vi "Keep Alive Interval.vi"(8 "error in (no error)":errorcluster, 9 "Connection Name":string, 11 "Keep Alive Interval (s)":i32) -> (0 "error out":errorcluster)   [LabVIEW 2018, in "LabSFTP.lvlib"]
doc: "<License>This software is distributed under the BSD 3-Clause License. For the full license please see license.txt or visit www.labvolution.com/license</License>"
uses:
  LabSFTP.lvlib
  FGV State..enum.ctl
  Z:/work/git/fpganow/MicroBlaze_lwIP/labview_fpga_nic/References/References/LabSFTP.dll
  References/LabSFTP.dll
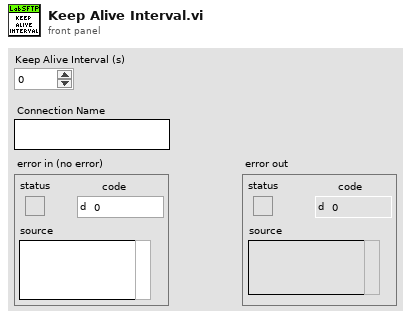
[diagram p1: front panel]
types:
  T1 = typedef "LabSFTP.lvlib/FGV State..enum.ctl" = enum16{"GET", "SET"}
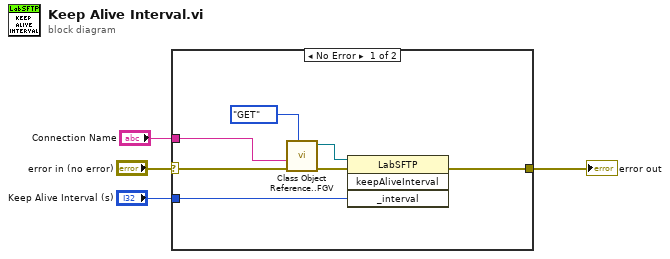
[diagram p0: block diagram]
diagram:
  n1 = case shown="No Error" "error in (no error)" {
    selector: "error in (no error)" -> [w8 w12]
    tunnel: [w7 w12] -> w4
    tunnel: "Keep Alive Interval (s)" -> [w6 _]
    tunnel: "Connection Name" -> [w5 _]
    frame No Error {
      n2 = call "Class Object Reference..FGV.vi"("FGV State"=FGV_State..enum."GET", "error in (no error)"=w8, "Connection Name"=w5) -> ("error out"=w9:errorcluster, "LabSFTP ref out"=w10:refnum<k24>)  [unwired: 7 in]
      n3 = invoke on="Invoke Node" class="LabSFTP" method="keepAliveInterval"(reference=w10, error in=w9, "_interval"=w6) -> (error out=w7:errorcluster)  [unwired: 1 in, 3 out]
    }
    frame Error {
    }
  }
  "error out" <- w4
